vi "Manuscript Bioreactor Labview.vi"() -> ()   [LabVIEW 2017]
doc: "Demonstrates how the Move Sin VI can be used to easily set-up and run a sinusoidal motion. This example also records the position and displays a position vs time chart during the motion."
uses:
  <vilib>/DAQmx/read.llb/DAQmx Read (Analog 2D DBL NChan NSamp).vi
  <vilib>/DAQmx/miscellaneous.llb/DAQmx Fill In Error Info.vi
  Zaber A Series/Zaber A Series.lvlib
panel:
  in  "Filename":path=path "C:/Users/kup225/Desktop/save/test save.lvm"
  out "Motor position":cluster{dbl[], dbl[]}(graph)
  in  "Total Hours to Run":dbl
  in  "Period in milliseconds":dbl=0.2 min=0.2 step=0.1 format="%#.1f"
  in  "Amplitude (mm) (half of peak - peak)":dbl
  in  "VISA resource name":refnum<visa-resource-name>
  in  "?":bool
  out "LVDT 1":cluster{dbl[], dbl[]}(graph)
  out "Load":cluster{dbl[], dbl[]}(graph)
  out "LVDT 2":cluster{dbl[], dbl[]}(graph)
  out "LVDT 3":cluster{dbl[], dbl[]}(graph)
  out "LVDT 4":cluster{dbl[], dbl[]}(graph)
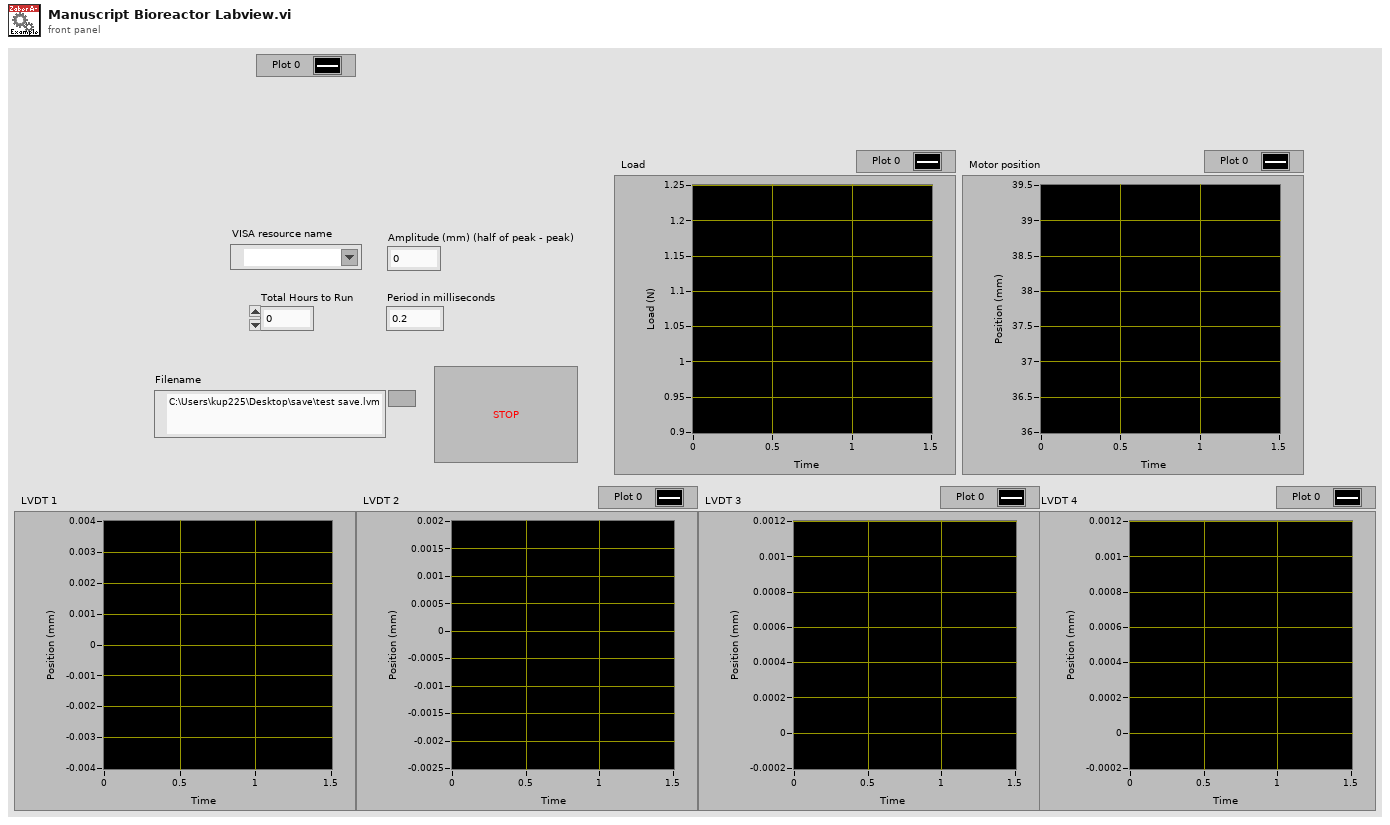
[diagram p1: front panel]
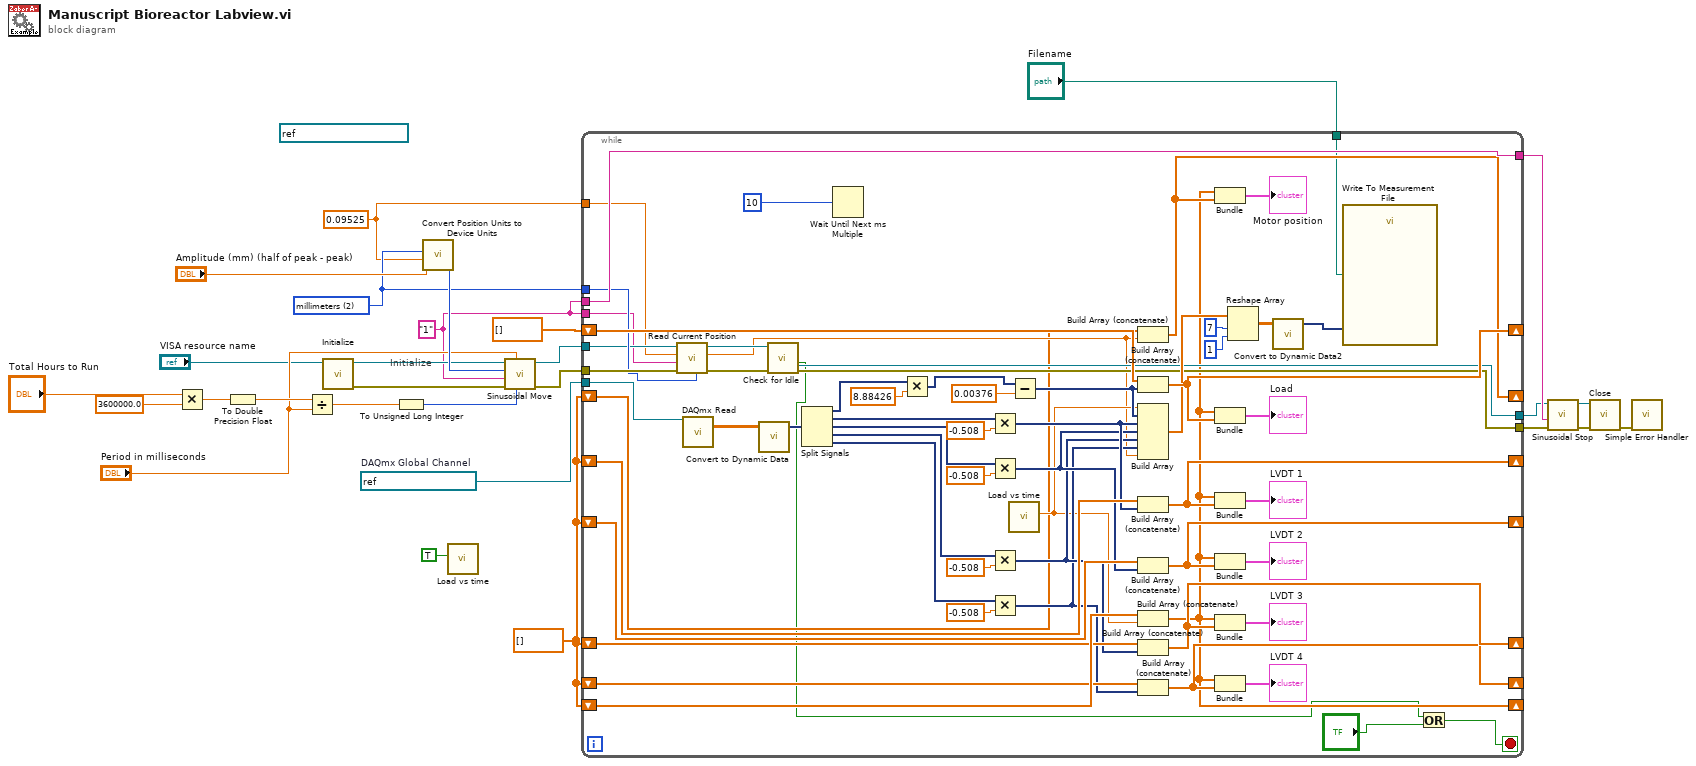
[diagram p0: block diagram]
diagram:
  (unwired) refnum<k21> "MyVoltageChannel"
  w3 = refnum<k21> "load cell, lvdt 1:4"  # DAQmx Global Channel
  w7 = "1" ("Device and Axis")
  w9 = u16 2 items=["microsteps", "microns", "millimeters", "inches", "degrees"] ("Units (0: microsteps) 2")
  w6 = 0.09525 ("Microstep Size (0)")
  w4 = dbl[] []
  # "Initialize"
  n1 = Multiply(x="Total Hours to Run", y=3600000.0) -> (x*y=w2:dbl)
  n2 = To Double Precision Float(number=w2) -> (double precision float=w17:dbl)
  n3 = Divide(x=w17, y="Period in milliseconds") -> (x/y=w16:dbl)
  n4 = call "Initialize.vi"("VISA resource name"="VISA resource name") -> ("error out"=w11:errorcluster, "VISA resource name out"=w12:refnum<visa-resource-name>)  [unwired: 9 in]
  n5 = To Unsigned Long Integer(number=w16) -> (unsigned 32bit integer=w15:u32)
  n6 = call "Convert Position Units to Device Units.vi"("Microstep Size (0)"=w6, "Units (0: microsteps)"=w9, "Position (0)"="Amplitude (mm) (half of peak - peak)") -> ("Device Position (32-bit)"=w20:i32)  [unwired: 6 in, 2 out]
  n7 = call "Load vs time.vi"("Reset"=TRUE) -> ()  [unwired: 9 in, 1 out]
  n8 = call "Sinusoidal Move.vi"("Cycle Count (0)"=w15, "Period"="Period in milliseconds", "error in (no error)"=w11, "Device and Axis"=w7, "Amplitude"=w20, "VISA resource name"=w12) -> ("error out"=w10:errorcluster, "VISA resource name out"=w8:refnum<visa-resource-name>)  [unwired: 4 in]
  n9 = while {
    shift-right: [w38] -> _
    shift-left: w4 -> [w83]
    shift-right: [w90] -> _
    shift-left: w4 -> [w73]
    tunnel: w3 -> [w89]
    shift-right: [w85] -> _
    shift-left: dbl[] [] -> [w84]
    shift-right: [w70] -> _
    shift-left: w4 -> [w71]
    shift-right: [w68] -> _
    shift-left: w4 -> [w69]
    shift-right: [w66] -> _
    shift-left: w4 -> [w67]
    tunnel: [w47] -> w23
    tunnel: [w46] -> w22
    tunnel: w7 -> [w46]
    tunnel: w10 -> [w45]
    tunnel: w9 -> [w44]
    tunnel: w8 -> [w43]
    tunnel: w7 -> [w42]
    tunnel: w6 -> [w41]
    tunnel: [w40] -> w5
    shift-right: [w39] -> _
    shift-left: w4 -> [w35]
    tunnel: "Filename" -> [w30]
    stop <- w32 stop-if-true
    n10 = call "Read Current Position.vi"("Units (0: microsteps)"=w44, "error in (no error)"=w45, "Device and Axis"=w42, "Microstep Size (0)"=w41, "VISA resource name"=w43) -> ("error out"=w48:errorcluster, "Position"=w36:dbl, "VISA resource name out"=w49:refnum<visa-resource-name>)  [unwired: 4 in]
    n11 = call-poly <vilib>:"DAQmx Read.vi"("task/channels in"=w89) -> ("data"=w87:dbl[][])  [unwired: 12 in, 2 out]
    n12 = call "Convert to Dynamic Data"("2D Array"=w87) -> ("Dynamic Data Type"=w86:dynamicdata)  [unwired: 3 in]
    n13 = call "Check for Idle.vi"("error in (no error)"=w48, "VISA resource name"=w49) -> ("error out"=w47:errorcluster, "Idle"=w34:bool, "VISA resource name out"=w40:refnum<visa-resource-name>)  [unwired: 7 in]
    n14 = Split Signals(w86) -> (w64:dynamicdata, w63:dynamicdata, w62:dynamicdata, w61:dynamicdata, w58:dynamicdata)  [unwired: 5 in]
    n15 = Wait Until Next ms Multiple(millisecond multiple=u32 10) -> ()  [unwired: 1 out]
    n16 = Multiply(x=w64, y=8.88426) -> (x*y=w81:dynamicdata)
    n17 = Multiply(x=w63, y=-0.508) -> (x*y=w55:dynamicdata)
    n18 = Multiply(x=w62, y=-0.508) -> (x*y=w54:dynamicdata)
    n19 = Multiply(x=w61, y=-0.508) -> (x*y=w53:dynamicdata)
    n20 = Multiply(x=w58, y=-0.508) -> (x*y=w52:dynamicdata)
    n21 = call "Load vs time.vi"() -> ("Time(s)"=w51:dbl)  [unwired: 10 in]
    n22 = Subtract(x=w81, y=0.00376) -> (x-y=w56:dynamicdata)
    n23 = Build Array (concatenate)(w35, w36) -> (w39:dbl[])
    n24 = Build Array (concatenate)(w84, w56) -> (w85:dbl[])
    n25 = Build Array(w51, w56, w55, w54, w53, w52, w36) -> (w50:dbl[])
    n26 = Build Array (concatenate)(w73, w55) -> (w90:dbl[])
    n27 = Build Array (concatenate)(w71, w54) -> (w70:dbl[])
    n28 = Build Array (concatenate)(w83, w51) -> (w38:dbl[])
    n29 = Build Array (concatenate)(w69, w53) -> (w68:dbl[])
    n30 = Build Array (concatenate)(w67, w52) -> (w66:dbl[])
    n31 = Bundle(w38, w39) -> (→"Motor position":cluster{dbl[], dbl[]})  [unwired: 1 in]
    n32 = Bundle(w38, w85) -> (→"Load":cluster{dbl[], dbl[]})  [unwired: 1 in]
    n33 = Bundle(w38, w90) -> (→"LVDT 1":cluster{dbl[], dbl[]})  [unwired: 1 in]
    n34 = Bundle(w38, w70) -> (→"LVDT 2":cluster{dbl[], dbl[]})  [unwired: 1 in]
    n35 = Bundle(w38, w68) -> (→"LVDT 3":cluster{dbl[], dbl[]})  [unwired: 1 in]
    n36 = Bundle(w38, w66) -> (→"LVDT 4":cluster{dbl[], dbl[]})  [unwired: 1 in]
    n37 = Reshape Array(w50, 7 ("dimension size"), 1 ("dimension size")) -> (w57:dbl[][])
    n38 = call "Convert to Dynamic Data2"("2D Array"=w57) -> ("Dynamic Data Type"=w31:dynamicdata)  [unwired: 3 in]
    n39 = call "Write To Measurement File"("Signals"=w31, "Filename"=w30) -> ()  [unwired: 15 in, 3 out]
    n40 = Or(x=w34, y="?") -> (x .or. y?=w32:bool)
  }
  n41 = call "Sinusoidal Stop.vi"("error in (no error)"=w23, "Device and Axis"=w22, "VISA resource name"=w5) -> ("error out"=w24:errorcluster, "VISA resource name out"=w25:refnum<visa-resource-name>)  [unwired: 7 in]
  n42 = call "Close.vi"("error in (no error)"=w24, "VISA resource name"=w25) -> ("error out"=w26:errorcluster)  [unwired: 9 in]
  n43 = call <vilib>:"Simple Error Handler.vi"("error in (no error)"=w26) -> ()  [unwired: 4 in, 5 out]
